vi "Siren Test.vi"() -> ()   [LabVIEW 2012]
panel:
  in  "Stop":bool
  in  "Active":bool
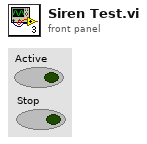
[diagram p1: front panel]
types:
  T1 = typedef "Sound Output Task ID.ctl" = u32
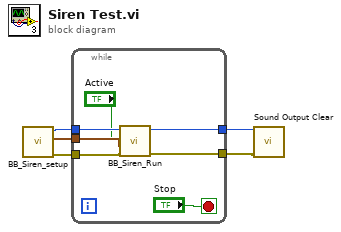
[diagram p0: block diagram]
diagram:
  n1 = call "BB_Siren_setup.vi"() -> ("error out"=w3:errorcluster, "Sampling Info"=w4:cluster{"Fs":dbl, "#s":dbl}, "task ID"=w5:T1)  [unwired: 9 in]
  n2 = while {
    tunnel: w5 -> [w11]
    tunnel: w4 -> [w10]
    tunnel: w3 -> [w8]
    tunnel: [w7] -> w2
    tunnel: [w6] -> w1
    stop <- "Stop" stop-if-true
    n3 = call "BB_Siren_Run.vi"("Error In"=w8, "sampling info"=w10, "Active"="Active", "Task ID In"=w11) -> ("error out"=w7:errorcluster, "task ID out"=w6:T1)  [unwired: 6 in]
  }
  n4 = call <vilib>:"Sound Output Clear.vi"("error in (no error)"=w2, "task ID"=w1) -> ()  [unwired: 9 in, 1 out]
